vi "Set Inputs.vi"(10 "Inputs":dbl[](array[numeric]), 11 "AER in":refnum<class "AER.lvclass">) -> (3 "AER out":refnum<class "AER.lvclass">)   [LabVIEW 2016, in "AER.lvclass"]
doc: "This Vi updates the currents of the mfs from distributing the inputs"
uses:
  AER.lvclass
  Controls/Type of Neuron.ctl
  AER.lvclass/AER.ctl
panel:
  out "W":dbl[](graph)
  out "size W":i32
  out "size Currents":i32
  out "No MFs":i32
  out "Firing rates":dbl[](graph)
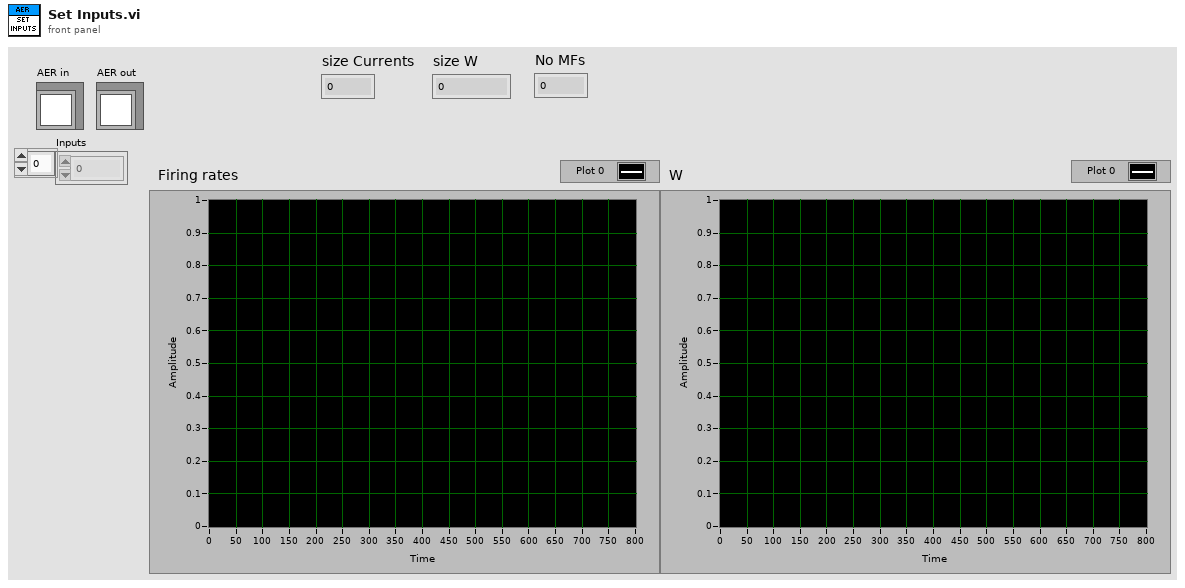
[diagram p1: front panel]
types:
  T1 = typedef "Type of Neuron.ctl" = enum16{"MF", "BA", "GO", "GC", "PC", "LU", "Glia (Dummy)"}
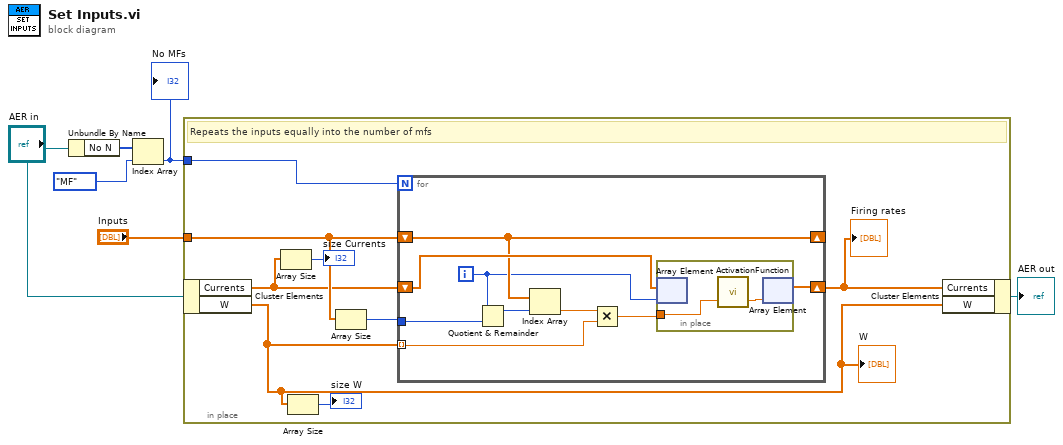
[diagram p0: block diagram]
diagram:
  n1 = Unbundle By Name("AER in") -> ("No N"=w3:i32[])
  n2 = Index Array(array=w3, index=Type_of_Neuron."MF" ("Type of Neuron")) -> (element=w2:i32)
  "No MFs" <- w2
  n3 = in-place {
    in-place-border: "Inputs" -> [w13]
    in-place-border: w2 -> [w14]
    # "Repeats the inputs equally into the number of mfs"
    n4 = in-place-cluster #1("AER in") -> ("Currents"=w10:dbl[], "W"=w7:dbl[])
    "W" <- w7
    n5 = Array Size(array=w10) -> (size(s)=→"size Currents":i32)
    n6 = Array Size(array=w7) -> (size(s)=→"size W":i32)
    n7 = Array Size(array=w13) -> (size(s)=w12:i32)
    n8 = for {
      N: w14 -> [_]
      shift-right: [w20] -> w11
      shift-left: w10 -> [w22]
      tunnel: w12 -> [w19]
      tunnel: w7 -> [w15] mode=indexing
      shift-right: [w18] -> _
      shift-left: w13 -> [w18]
      i -> [w16]
      n9 = Quotient & Remainder(x=w16, y=w19) -> (x-y*floor(x/y)=w17:i32)  [unwired: 1 out]
      n10 = Index Array(array=w18, index=w17) -> (element=w23:dbl)
      n11 = Multiply(x=w23, y=w15) -> (x*y=w21:dbl)
      n12 = in-place {
        in-place-border: w21 -> [w25]
        n13 = in-place-array #2(w22, w16) -> ()  [unwired: 1 out]
        n14 = call "ActivationFunction.vi"("x"=w25) -> ("y"=w24:dbl)  [unwired: 2 in]
        n15 = in-place-array #2(w24) -> (w20:dbl[])  [unwired: 1 out]
      }
    }
    "Firing rates" <- w11
    n16 = in-place-cluster #1("Currents"=w11, "W"=w7) -> (→"AER out":refnum<class "AER.lvclass">)
  }
